vi "LWXPS_CIERegisterValueSet.vi"(0 "XPS Reference IN":refnum<k24>, 5 "Positioner Name":string, 7 "Board Offset":i16, 9 "Register Value":i32, 11 "LabVIEW error IN":errorcluster caption="error LabVIEW error IN") -> (4 "XPS Reference OUT":refnum<k24>, 6 "Returned error code":i32, 10 "XPS Error String":string, 15 "LabVIEW error OUT":errorcluster)   [LabVIEW 2014]
uses:
  D:/XPSQ8_LabView_Library/Development/Source/Dll/Newport.XPS.CommandInterface.dll
  Dll/Newport.XPS.CommandInterface.dll
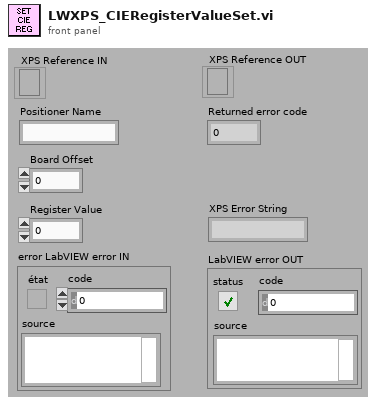
[diagram p1: front panel]
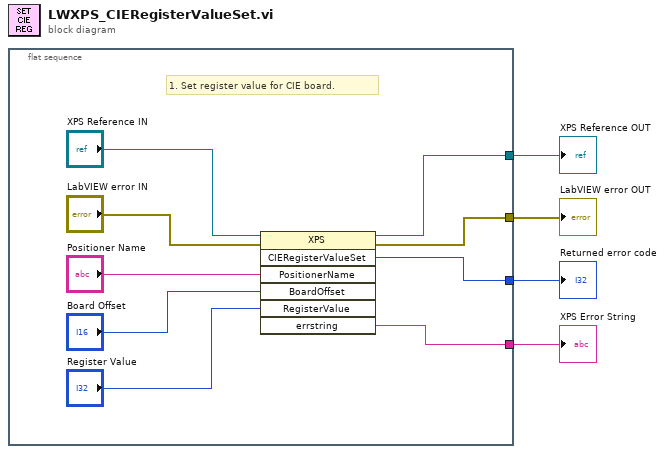
[diagram p0: block diagram]
diagram:
  n1 = flat-sequence {
    tunnel: [w6] -> w4
    tunnel: [w11] -> w3
    tunnel: [w7] -> w2
    tunnel: [w10] -> w1
    frame #0 {
      # "1. Set register value for CIE board."
      n2 = invoke class="XPS" method="CIERegisterValueSet"(reference="XPS Reference IN", error in="LabVIEW error IN", "PositionerName"="Positioner Name", "BoardOffset"="Board Offset", "RegisterValue"="Register Value") -> (reference out=w6:refnum<k24>, error out=w11:errorcluster, "CIERegisterValueSet"=w10:i32, "errstring"=w7:string)  [unwired: 2 in, 3 out]
    }
  }
  "XPS Reference OUT" <- w4
  "LabVIEW error OUT" <- w3
  "XPS Error String" <- w2
  "Returned error code" <- w1
